vi "Read Temperature.vi"(8 "error in (no error)":errorcluster, 11 "Grove Thermocouple MCP9600 in":refnum<class "Grove Thermocouple MCP9600.lvclass">) -> (0 "error out":errorcluster, 2 "Temperature":dbl, 3 "Grove Thermocouple MCP9600 out":refnum<class "Grove Thermocouple MCP9600.lvclass">)   [LabVIEW 2020, in "CTI-Peripheral.lvlib" / "Grove Thermocouple MCP9600.lvclass"]
uses:
  Grove Thermocouple MCP9600.lvclass
  Grove Thermocouple MCP9600.lvclass/Grove Thermocouple MCP9600.ctl
  CTI/I2C Connection/I2C Connection.lvclass/I2C Connection.ctl
  CTI/Session/I2C Write Data.vi
  CTI/Session/I2C Read Data.vi
  CTI/I2C Connection/I2C Connection.lvclass
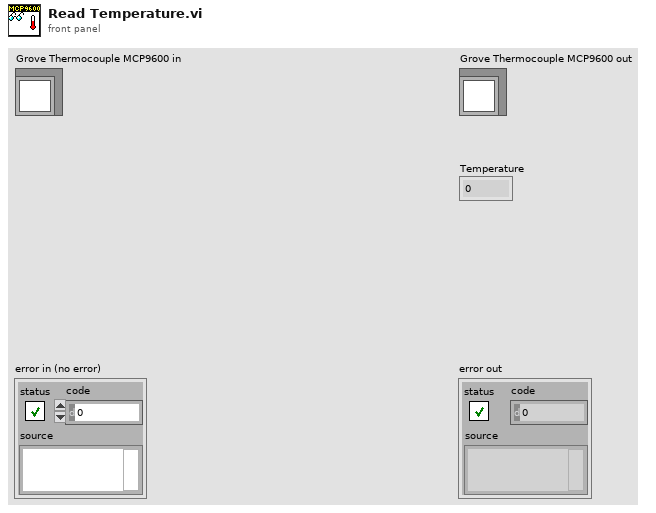
[diagram p1: front panel]
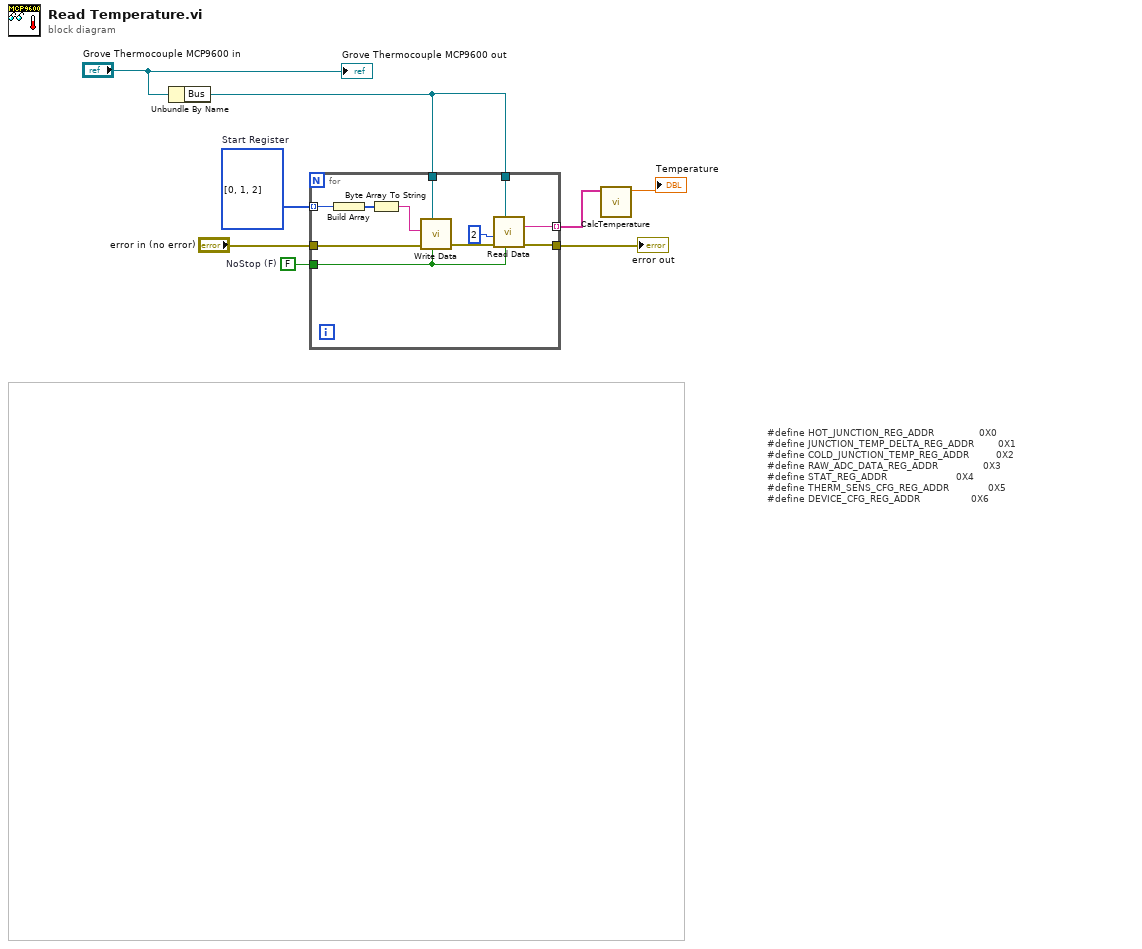
[diagram p0: block diagram]
diagram:
  w7 = u8[] [0, 1, 2]  # Start Register
  w3 = FALSE  # NoStop (F)
  # "#define HOT_JUNCTION_REG_ADDR               0X0\n#define JUNCTION_TEMP_DELTA_REG_ADDR        0X1\n#define COLD_JUNCTION_TEMP_REG_ADDR         0X2\n#define RAW_ADC_DATA_REG_ADDR               0X3\n#define STAT_REG_ADDR                       0X4\n#define THERM_SENS_CFG_REG_ADDR             0X5\n#define DEVICE_CFG_REG_ADDR                 0X6"
  n1 = Unbundle By Name("Grove Thermocouple MCP9600 in") -> ("Bus"=w4:refnum<class "I2C Connection.lvclass">)
  n2 = for {
    tunnel: w7 -> [w19] mode=indexing
    tunnel: [w16] -> w6
    tunnel: [w13] -> w2 mode=indexing
    tunnel: "error in (no error)" -> [w12]
    tunnel: w4 -> [w11]
    tunnel: w4 -> [w10]
    tunnel: w3 -> [w9]
    n3 = Build Array(w19) -> (w18:u8[])
    n4 = Byte Array To String(unsigned byte array=w18) -> (string=w15:string)
    n5 = call "Write Data.vi"("NoStop (F)"=w9, "I2C Connection"=w11, "error in (no error)"=w12, "Data"=w15) -> ("error out"=w17:errorcluster)  [unwired: 7 in]
    n6 = call "Read Data.vi"("NoStop (F)"=w9, "I2C Connection"=w10, "error in (no error)"=w17, "Len"=u8 2 ("Read Len")) -> ("error out"=w16:errorcluster, "Data"=w13:string)  [unwired: 6 in]
  }
  "error out" <- w6
  n7 = call "CalcTemperature.vi"("Array"=w2) -> ("HJ Temperature (°C)"=→"Temperature":dbl)  [unwired: 10 in]
  "Grove Thermocouple MCP9600 out" <- "Grove Thermocouple MCP9600 in"
